vi "DHFL1dll.vi"(8 "error in (no error)":errorcluster, 11 "Inputs":cluster{"d":dbl, "h":dbl, "z":dbl[], "t":dbl}) -> (0 "error out":errorcluster, 3 "Outputs":T1)   [LabVIEW 2015]
doc: "SINGLE-PHASE FLASH SUBROUTINES\n\nsubroutine DHFL1dll(d, h, z, t, ierr, herr, herr_length)\n\nThese routines accept only single-phase states as inputs. They will be\nfaster than the corresponding general routines, but will fail if called\nwith an incorrect phase specification. The phase-specific subroutines\nalso do not check limits, so may fail if called outside the range of the\nequation of state. The following single-phase routines are available.\n\nINPUTS: \nd -- molar density [mol/L]\nh -- enthalpy [J/mol]\nz -- overall (bulk) composition [array of mol frac]\nt -- temperature [K]\n\nOUTPUTS:\nt -- temperature [K] (present only for HSFL1)\nd -- molar density [mol/L]\nierr -- error flag: 0 = successful\nherr -- error string (character*255 variable if ierr<>0)\nherr_length -- length of variable herr (default: 255)"
uses:
  REFPROP.dll
panel:
  # "REFPROP-DHFL1.vi"
  # "void  DHFL1dll(double *d, double *h, double *z, double *t, int32_t *ierr, CStr herr, int32_t herr_length);"
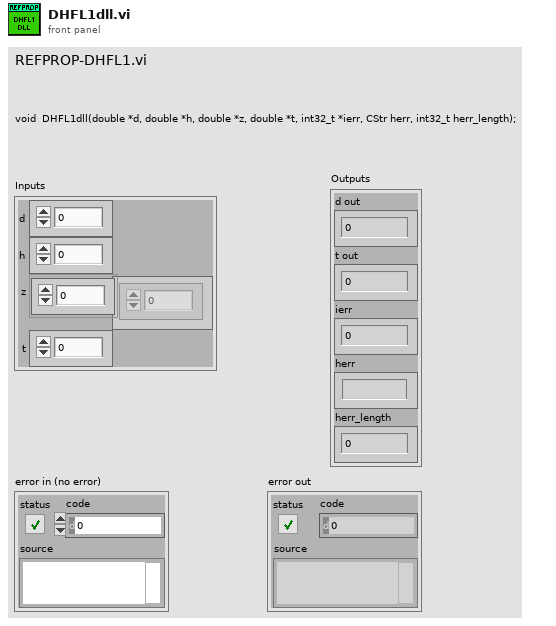
[diagram p1: front panel]
types:
  T1 = cluster{"d out":dbl, "t out":dbl, "ierr":i32, "herr ":string, "herr_length":i32}
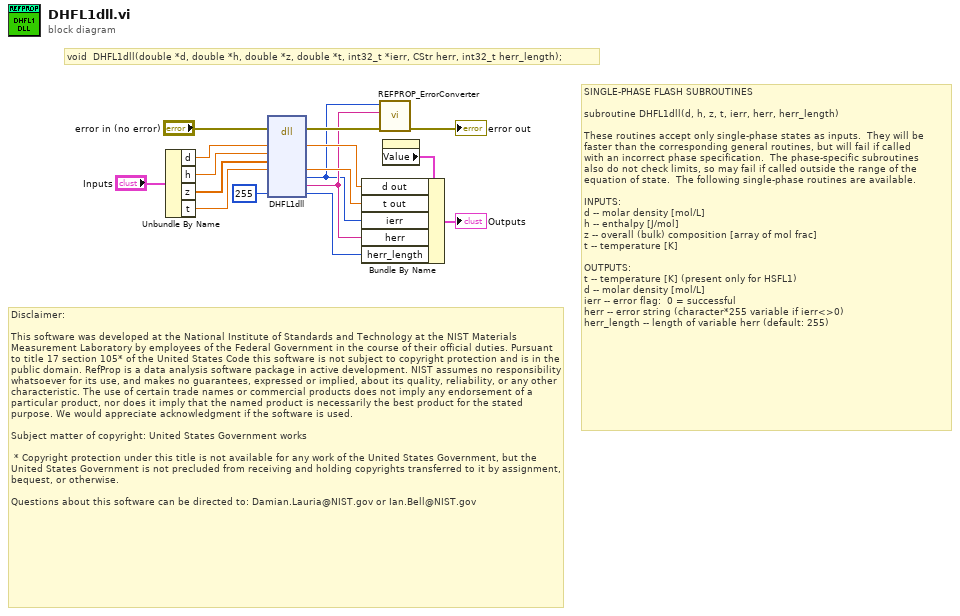
[diagram p0: block diagram]
diagram:
  # "Disclaimer:\n\nThis software was developed at the National Institute of Standards and Technology at the NIST Materials Measurement Laboratory by employees of the Federal Government in the course of their official duties. Pursuant to title 17 section 105* of the United States Code this software is not subject to copyright protection and is in the public domain. RefProp is a data analysis software package in active development. NIST assumes no responsibility whatsoever for its use, and makes no guarantees, expressed or implied, about its quality, reliability, or any other characteristic. The use of certain trade names or commercial products does not imply any endorsement of a particular product, nor does it imply that the named product is necessarily the best product for the stated purpose. We would appreciate acknowledgment if the software is used.\n \nSubject matter of copyright: United States Government works\n  \n * Copyright protection under this title is not available for any work of the United States Government, but the United States Government is not precluded from receiving and holding copyrights transferred to it by assignment, bequest, or otherwise.\n\nQuestions about this software can be directed to: Damian.Lauria@NIST.gov or Ian.Bell@NIST.gov"
  # "void  DHFL1dll(double *d, double *h, double *z, double *t, int32_t *ierr, CStr herr, int32_t herr_length);"
  # "SINGLE-PHASE FLASH SUBROUTINES\n\nsubroutine DHFL1dll(d, h, z, t, ierr, herr, herr_length)\n\nThese routines accept only single-phase states as inputs.  They will be\nfaster than the corresponding general routines, but will fail if called\nwith an incorrect phase specification.  The phase-specific subroutines\nalso do not check limits, so may fail if called outside the range of the\nequation of state.  The following single-phase routines are available.\n\nINPUTS: \nd -- molar density [mol/L]\nh -- enthalpy [J/mol]\nz -- overall (bulk) composition [array of mol frac]\nt -- temperature [K]\n\nOUTPUTS:\nt -- temperature [K] (present only for HSFL1)\nd -- molar density [mol/L]\nierr -- error flag:  0 = successful\nherr -- error string (character*255 variable if ierr<>0)\nherr_length -- length of variable herr (default: 255)"
  n1 = Unbundle By Name("Inputs") -> ("d"=w4:dbl, "h"=w3:dbl, "z"=w2:dbl[], "t"=w1:dbl)
  n2 = dll-call lib="C:/Users/lauria/Desktop/REFPROP 10 LabVIEW Wrapper BETA/REFPROP/REFPROP.*" fn="DHFL1dll"(error in="error in (no error)", "d"=w4, "h"=w3, "z"=w2, "t"=w1, "herr_length"=255 ("ln")) -> (error out=w15:errorcluster, "d"=w10:dbl, "t"=w9:dbl, "ierr"=w6:i32, "herr"=w7:string, "herr_length"=w8:i32)  [unwired: 7 in, 1 out]
  n3 = call "REFPROP_ErrorConverter.vi"("error in (no error)"=w15, "Error Message"=w7, "Error Code"=w6) -> ("error out"=→"error out":errorcluster)  [unwired: 8 in]
  n4 = property on="Outputs" class="Clust (strict)"() -> ("Value"=w11:T1)  [unwired: 2 in, 2 out]
  n5 = Bundle By Name(cluster=w11, "d out"=w10, "t out"=w9, "ierr"=w6, "herr"=w7, "herr_length"=w8) -> (→"Outputs":T1)
